vi "Add Injector.vi"(7 "Max Shots":T1(ring)=enum."1", 8 "error in (no error)":errorcluster, 9 "Stages":string[](array[string])=["Boost", "Battery", "Off"], 10 "Controls":T3[](array[typedef]) {"Data Type" format="%.0x"}, 11 "Item Ref":T2=18446744073709551615 format="%.0x") -> (0 "error out":errorcluster, 3 "Item Ref out":T2=18446744073709551615 format="%.0x")   [LabVIEW 2015, in "Fuel Injection Addon System Explorer.lvlib"]
uses:
  Fuel Injection Addon System Explorer.lvlib
  <vilib>/NI Veristand/Custom Device API/Custom Device Item Ref.ctl
  Shared/Types/Register.Info.ctl
  Shared/Types/FPGA Data Types.ctl
  FPGA IP/Types/Injection.Global.Settings.ctl
  Shared/Constants.vi
  <vilib>/NI Veristand/Custom Device API/Set Item Property (Variant).vi
  <vilib>/NI Veristand/Custom Device Tools/Custom Device Utility Library/NI VeriStand - Search for Item by GUID.vi
  Shared/Fuel Injection Addon Shared.lvlib
  <vilib>/NI VeriStand/Custom Device API/Custom Device API.lvlib
  <vilib>/NI Veristand/Custom Device Tools/Custom Device Utility Library/Custom Device Utility Library.lvlib
panel:
  in  "Tags":string
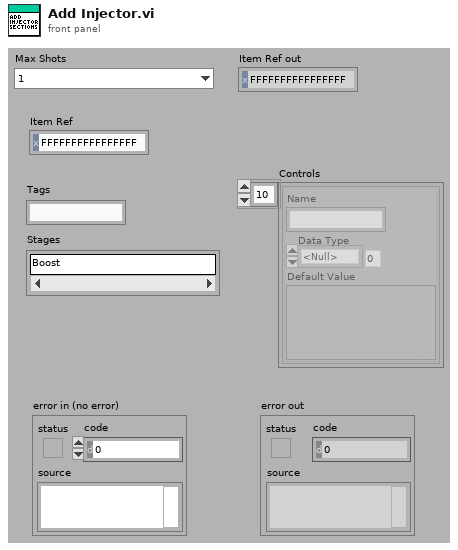
[diagram p1: front panel]
types:
  T1 = enum16{"0", "1", "2", "3", "4", "5", "6", "7", "8"}
  T2 = typedef "Custom Device API.lvlib/Custom Device Item Ref.ctl" = u64
  T3 = typedef "Fuel Injection Addon Shared.lvlib/Register.Info.ctl" = cluster{"Name":string, "Data Type":T4, "Default Value":variant}
  T4 = typedef "Fuel Injection Addon Shared.lvlib/FPGA Data Types.ctl" = enum8{"<Null>", "Injector.Core.Setting", "Injector.Global.Setting", "Injector.Mux.Setting", "Injector.Timing"}
  T5 = typedef "Injection.Global.Settings.ctl" = cluster{"Enable?":bool, "Initial Voltage Threshold":fxp<+/-,32,8>, "Remaining Voltage Threshold":fxp<+/-,32,8>, "Stage Dwell Limit":u16, "Event Dwell Limit":u16, "Voltage Gain":fxp<+/-,32,8>, "Current Gain":fxp<+/-,32,8>}
  T6 = cluster{"Voltage Offset":fxp<+/-,32,8>, "Current Offset":fxp<+/-,32,8>}
  T7 = typedef "Fuel Injection Addon Shared.lvlib/Main Settings.ctl" = cluster{"RIO Device Address":string, "Local bitfile path":path, "RT bitfile path":path, "Number of injectors":u16, "Max injection shot count":u16, "Sample rate (S/s)":u32, "Stages":string[]}
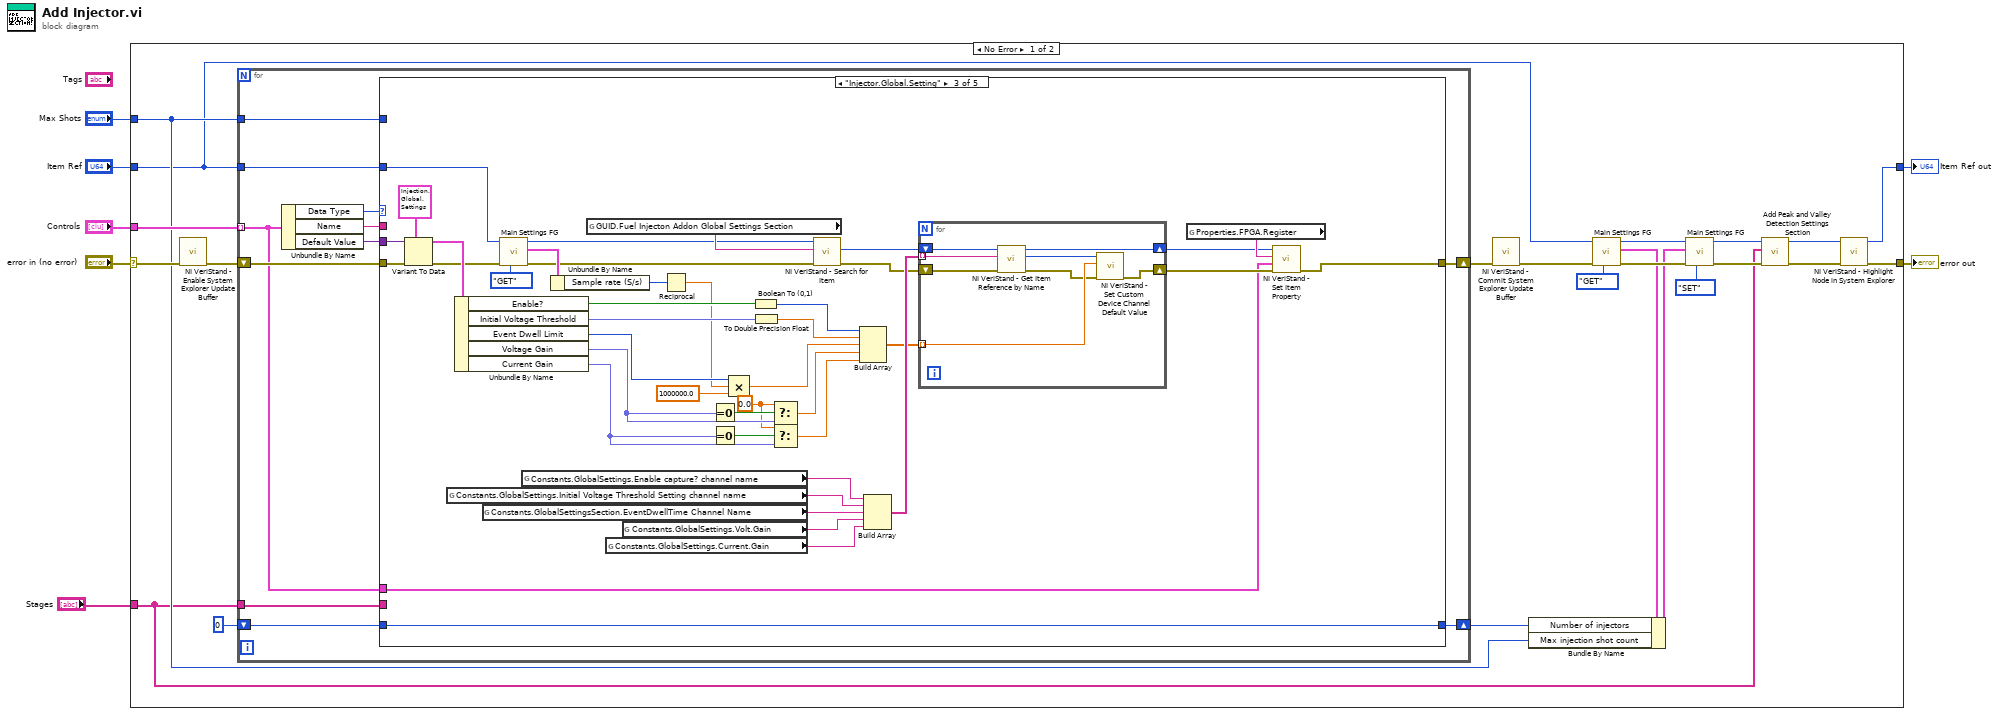
[diagram p0: block diagram]
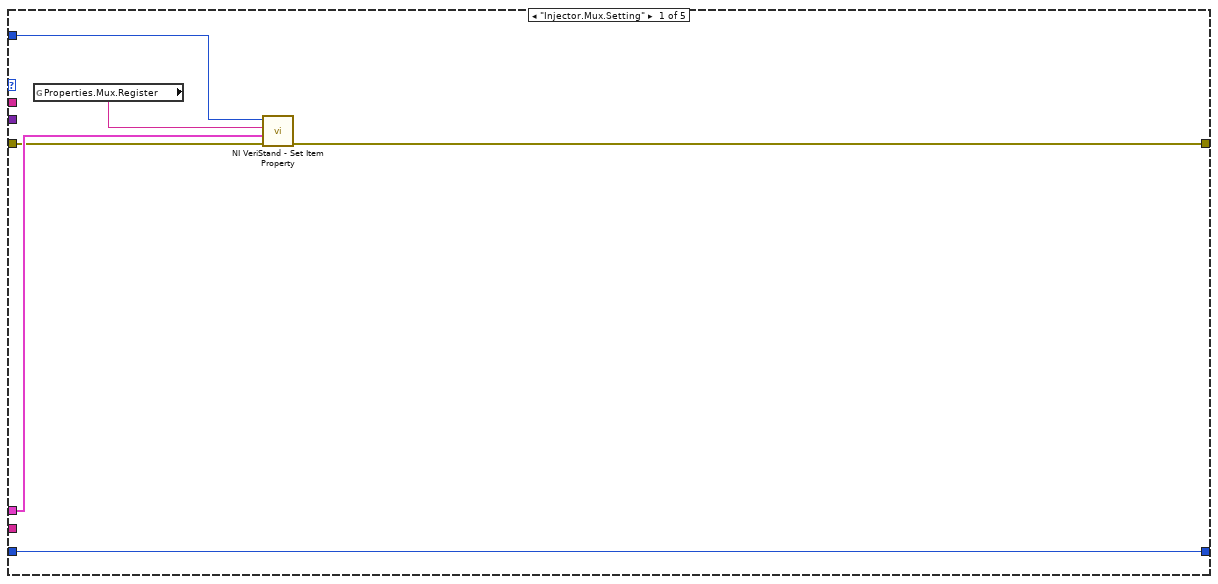
[diagram p2: hidden frame]
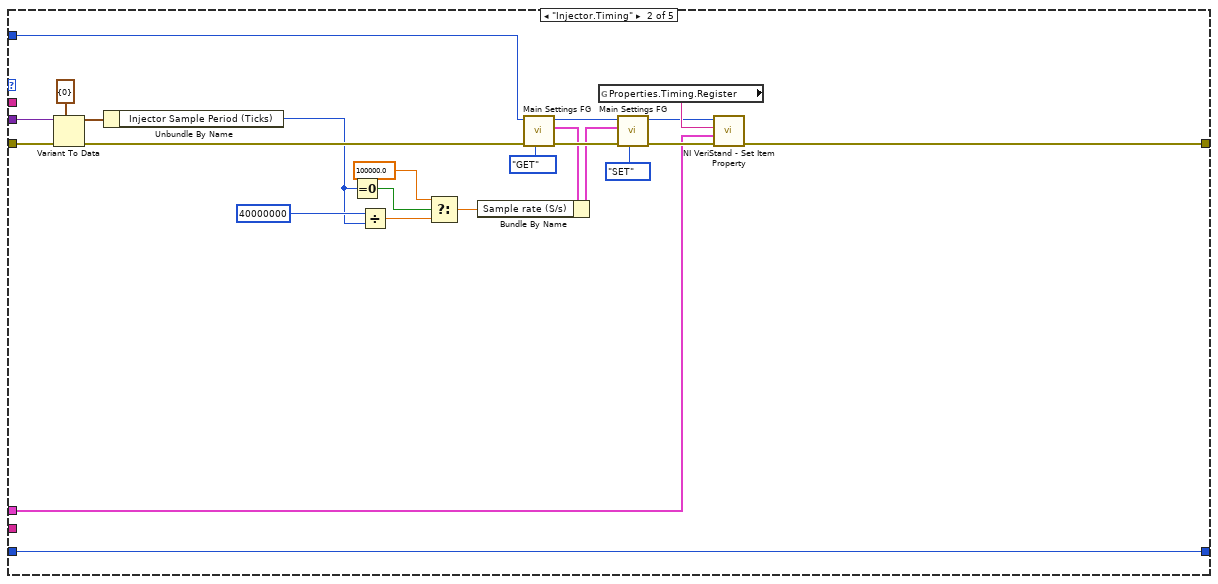
[diagram p3: hidden frame]
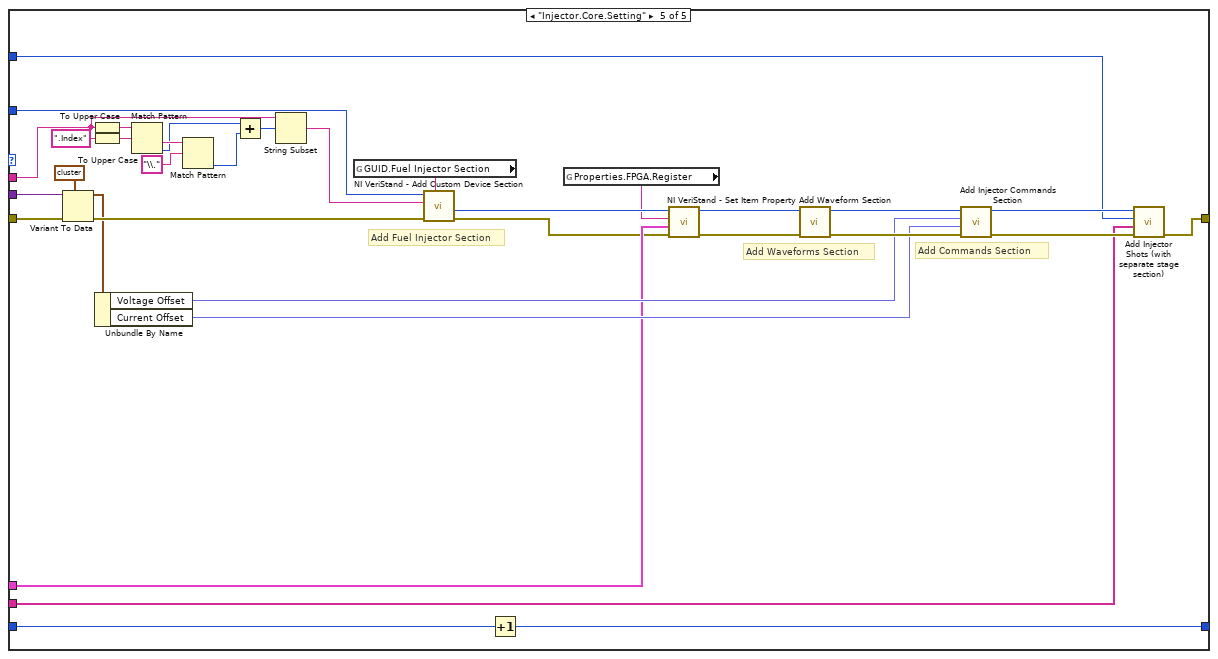
[diagram p5: hidden frame]
diagram:
  n1 = case shown="No Error" "error in (no error)" {
    selector: "error in (no error)" -> [w28 w158]
    tunnel: [w27 w158] -> w7
    tunnel: "Item Ref" -> [w16 w157]
    tunnel: "Controls" -> [w29 _]
    tunnel: [w26 w157] -> w3
    tunnel: "Stages" -> [w11 _]
    tunnel: "Max Shots" -> [w17 _]
    frame No Error {
      n2 = call <vilib>:"NI VeriStand - Enable System Explorer Update Buffer.vi"("error in (no error)"=w28) -> ("error out"=w15:errorcluster)  [unwired: 10 in]
      n3 = for {
        shift-right: [w39] -> w10
        shift-left: w15 -> [w40]
        tunnel: w29 -> [w37] mode=indexing
        shift-right: [w34] -> w18
        shift-left: u32 0 -> [w35]
        tunnel: w11 -> [w32]
        tunnel: w17 -> [w31]
        tunnel: w16 -> [w30]
        n4 = Unbundle By Name(w37) -> ("Data Type"=w33:T4, "Name"=w36:string, "Default Value"=w38:variant)
        n5 = case shown="\"Injector.Global.Setting\"" w33 {
          tunnel: w40 -> [w42 w63 w89 w122 w149]
          tunnel: [w41 w56 w85 w122 w151] -> w39
          tunnel: w30 -> [w43 w64 w88 _ w150]
          tunnel: w38 -> [_ w61 w112 _ w147]
          tunnel: w37 -> [w44 w52 w83 _ w138]
          tunnel: w36 -> [_ _ _ _ w130]
          tunnel: w35 -> [w46 w53 w82 w121 w137]
          tunnel: [w46 w53 w82 w121 w136] -> w34
          tunnel: w32 -> [_ _ _ _ w124]
          tunnel: w31 -> [_ _ _ _ w123]
          frame "Injector.Mux.Setting" {
            n6 = global read "Constants.vi" "Properties.Mux.Register"() -> (w45:string)
            n7 = call-poly <vilib>:"NI VeriStand - Set Item Property.vi"("error in (no error)"=w42, "Value"=w44, "Property Name"=w45, "Item Ref in"=w43) -> ("error out"=w41:errorcluster)  [unwired: 5 in, 2 out]
          }
          frame "Injector.Timing" {
            n8 = Variant To Data(error in=w63, type=cluster{"Injector Sample Period (Ticks)":u32} {"Injector Sample Period (Ticks)"=0} ("Injector.Timing"), Variant=w61) -> (data=w54:cluster{"Injector Sample Period (Ticks)":u32}, error out=w62:errorcluster)
            n9 = Unbundle By Name(w54) -> ("Injector Sample Period (Ticks)"=w51:u32)
            n10 = Equal To 0?(x=w51) -> (x = 0?=w50:bool)
            n11 = Divide(x=u32 40000000, y=w51) -> (x/y=w48:dbl)
            n12 = Select(t=100000.0, s=w50, f=w48) -> (s? t:f=w47:dbl)
            n13 = call "Main Settings FG.vi"("Action"=enum8{"GET", "SET"}."GET", "error in (no error)"=w62, "Item Ref"=w64) -> ("error out"=w70:errorcluster, "Main Settings out"=w69:T7, "Item Ref out"=w66:T2)  [unwired: 6 in]
            n14 = Bundle By Name(cluster=w69, "Sample rate (S/s)"=w47) -> (w68:T7)
            n15 = global read "Constants.vi" "Properties.Timing.Register"() -> (w58:string)
            n16 = call "Main Settings FG.vi"("Action"=enum8{"GET", "SET"}."SET", "error in (no error)"=w70, "Main Settings"=w68, "Item Ref"=w66) -> ("error out"=w57:errorcluster, "Item Ref out"=w55:T2)  [unwired: 5 in, 1 out]
            n17 = call-poly <vilib>:"NI VeriStand - Set Item Property.vi"("error in (no error)"=w57, "Value"=w52, "Property Name"=w58, "Item Ref in"=w55) -> ("error out"=w56:errorcluster)  [unwired: 5 in, 2 out]
          }
          frame "Injector.Global.Setting" {
            w76 = 0.0 ("x*y")
            n18 = Variant To Data(error in=w89, type=T5 {"Enable?"=FALSE, "Initial Voltage Threshold"=0.0, "Remaining Voltage Threshold"=12.0, "Stage Dwell Limit"=2000, "Event Dwell Limit"=0, "Voltage Gain"=0.0, "Current Gain"=1.0} ("InjectorAnalysis.Settings"), Variant=w112) -> (data=w111:T5, error out=w95:errorcluster)
            n19 = global read "Constants.vi" "Constants.GlobalSettings.Initial Voltage Threshold Setting channel name"() -> (w71:string)
            n20 = Unbundle By Name(w111) -> ("Enable?"=w101:bool, "Initial Voltage Threshold"=w102:fxp<+/-,32,8>, "Event Dwell Limit"=w91:u16, "Voltage Gain"=w80:fxp<+/-,32,8>, "Current Gain"=w74:fxp<+/-,32,8>)
            n21 = global read "Constants.vi" "Constants.GlobalSettingsSection.EventDwellTime Channel Name"() -> (w107:string)
            n22 = call "Main Settings FG.vi"("Action"=enum8{"GET", "SET"}."GET", "error in (no error)"=w95, "Item Ref"=w88) -> ("error out"=w94:errorcluster, "Main Settings out"=w97:T7, "Item Ref out"=w93:T2)  [unwired: 6 in]
            n23 = global read "Constants.vi" "Constants.GlobalSettings.Enable capture? channel name"() -> (w108:string)
            n24 = Unbundle By Name(w97) -> ("Sample rate (S/s)"=w92:u32)
            n25 = global read "Constants.vi" "GUID.Fuel Injecton Addon Global Settings Section"() -> (w109:string)
            n26 = global read "Constants.vi" "Constants.GlobalSettings.Current.Gain"() -> (w105:string)
            n27 = global read "Constants.vi" "Constants.GlobalSettings.Volt.Gain"() -> (w106:string)
            n28 = Reciprocal(x=w92) -> (1/x=w90:dbl)
            n29 = Equal To 0?(x=w80) -> (x = 0?=w81:bool)
            n30 = Equal To 0?(x=w74) -> (x = 0?=w77:bool)
            n31 = Compound Arithmetic op=MULTIPLY(w91, w90, 1000000.0 ("value")) -> (w78:dbl)
            n32 = Boolean To (0,1)(Boolean=w101) -> (0, 1=w100:i16)
            n33 = To Double Precision Float(number=w102) -> (double precision float=w99:dbl)
            n34 = Select(t=w76, s=w81, f=w80) -> (s? t:f=w79:dbl)
            n35 = Select(t=w76, s=w77, f=w74) -> (s? t:f=w75:dbl)
            n36 = call-poly <vilib>:"NI VeriStand - Search for Item.vi"("error in"=w94, "Item GUID"=w109, "Section Ref in"=w93) -> ("error out"=w103:errorcluster, "Item Ref"=w72:T2)  [unwired: 5 in, 2 out]
            n37 = Build Array(w100, w99, w78, w79, w75) -> (w98:dbl[])
            n38 = Build Array(w108, w71, w107, w106, w105) -> (w104:string[])
            n39 = for {
              tunnel: w104 -> [w117] mode=indexing
              shift-right: [w120] -> w86
              shift-left: w103 -> [w116]
              tunnel: w98 -> [w119] mode=indexing
              shift-right: [w114] -> w84
              shift-left: w72 -> [w118]
              n40 = call <vilib>:"NI VeriStand - Get Item Reference by Name.vi"("error in (no error)"=w116, "Item Name"=w117, "Parent Ref in"=w118) -> ("error out"=w115:errorcluster, "Item Ref"=w113:T2, "Parent Ref out"=w114:T2)  [unwired: 5 in, 1 out]
              n41 = call <vilib>:"NI VeriStand - Set Custom Device Channel Default Value.vi"("error in (no error)"=w115, "Default Value"=w119, "Channel Ref in"=w113) -> ("error out"=w120:errorcluster)  [unwired: 7 in, 1 out]
            }
            n42 = global read "Constants.vi" "Properties.FPGA.Register"() -> (w87:string)
            n43 = call-poly <vilib>:"NI VeriStand - Set Item Property.vi"("error in (no error)"=w86, "Value"=w83, "Property Name"=w87, "Item Ref in"=w84) -> ("error out"=w85:errorcluster)  [unwired: 5 in, 2 out]
          }
          frame "<Null>", Default {
          }
          frame "Injector.Core.Setting" {
            # "Add Commands Section"
            # "Add Waveforms Section"
            # "Add Fuel Injector Section"
            n44 = Variant To Data(error in=w149, type=T6 {"Voltage Offset"=0.0, "Current Offset"=0.0} ("Injector.Core.Settings Ch5"), Variant=w147) -> (data=w145:T6, error out=w148:errorcluster)
            n45 = To Upper Case(1:w130) -> (0:w134:string)
            n46 = To Upper Case(1:".Index" ("regular expression")) -> (0:w133:string)
            n47 = Unbundle By Name(w145) -> ("Voltage Offset"=w144:fxp<+/-,32,8>, "Current Offset"=w143:fxp<+/-,32,8>)
            n48 = Match Pattern(string=w134, regular expression=w133) -> (after substring=w132:string, offset past match=w128:i32)  [unwired: 1 in, 2 out]
            n49 = Match Pattern(string=w132, regular expression="\\.") -> (offset past match=w127:i32)  [unwired: 1 in, 3 out]
            n50 = Add(x=w128, y=w127) -> (x+y=w126:i32)
            n51 = String Subset(string=w130, offset (0)=w126) -> (substring=w129:string)  [unwired: 1 in]
            n52 = global read "Constants.vi" "GUID.Fuel Injector Section"() -> (w154:string)
            n53 = call <vilib>:"NI VeriStand - Add Custom Device Section.vi"("GUID (Default Section)"=w154, "error in (no error)"=w148, "Section Name"=w129, "Parent Ref in"=w150) -> ("error out"=w125:errorcluster, "Section Ptr"=w140:T2)  [unwired: 4 in, 2 out]
            n54 = Increment(x=w137) -> (x+1=w136:u32)
            n55 = global read "Constants.vi" "Properties.FPGA.Register"() -> (w139:string)
            n56 = call-poly <vilib>:"NI VeriStand - Set Item Property.vi"("error in (no error)"=w125, "Value"=w138, "Property Name"=w139, "Item Ref in"=w140) -> ("error out"=w142:errorcluster, "Item Ref out"=w141:T2)  [unwired: 5 in, 1 out]
            n57 = call "Add Waveform Section.vi"("error in (no error)"=w142, "Section Ptr"=w141) -> ("error out"=w156:errorcluster, "Injector Section ptr"=w155:T2)  [unwired: 8 in]
            n58 = call "Add Injector Commands Section.vi"("error in (no error)"=w156, "Default Current Offset"=w143, "Default Volt Offset"=w144, "Injector Section ptr"=w155) -> ("error out"=w152:errorcluster, "Parent Ref out"=w153:T2)  [unwired: 6 in]
            n59 = call "Add Injector Shots (with separate stage section).vi"("error in (no error)"=w152, "Stage Names"=w124, "# shots to add"=w123, "Injector Section Ref in"=w153) -> ("error out"=w151:errorcluster)  [unwired: 7 in]
          }
        }
      }
      n60 = call <vilib>:"NI VeriStand - Commit System Explorer Update Buffer.vi"("error in (no error)"=w10) -> ("error out"=w9:errorcluster)  [unwired: 10 in]
      n61 = call "Main Settings FG.vi"("Action"=enum8{"GET", "SET"}."GET", "error in (no error)"=w9, "Item Ref"=w16) -> ("error out"=w25:errorcluster, "Main Settings out"=w24:T7, "Item Ref out"=w21:T2)  [unwired: 6 in]
      n62 = Bundle By Name(cluster=w24, "Number of injectors"=w18, "Max injection shot count"=w17) -> (w23:T7)
      n63 = call "Main Settings FG.vi"("Action"=enum8{"GET", "SET"}."SET", "error in (no error)"=w25, "Main Settings"=w23, "Item Ref"=w21) -> ("error out"=w14:errorcluster, "Item Ref out"=w13:T2)  [unwired: 5 in, 1 out]
      n64 = call "Add Peak and Valley Detection Settings Section.vi"("error in (no error)"=w14, "Stages"=w11, "Global Settings Item Ref in"=w13) -> ("error out"=w8:errorcluster, "Global Settings Item Ref out"=w12:T2)  [unwired: 7 in]
      n65 = call <vilib>:"NI VeriStand - Highlight Node in System Explorer.vi"("error in (no error)"=w8, "Item Ref in"=w12) -> ("error out"=w27:errorcluster, "Node Ptr dup"=w26:T2)  [unwired: 8 in]
    }
    frame Error {
    }
  }
  "error out" <- w7
  "Item Ref out" <- w3
